vi "Initialize Tasks - NTask.vi"(6 "initialize and close session behavior":T1, 7 "option string":string, 8 "error in":errorcluster, 9 "reset":bool, 11 "session reservation in":refnum<class "Session Reservation.lvclass">) -> (0 "error out":errorcluster, 1 "channel lists":string[](array[string]), 2 "tasks":refnum<class "Session Factory.lvclass">[](array[class]), 3 "session reservation out":refnum<class "Session Reservation.lvclass">)   [LabVIEW 2021, in "Session Management niDAQmx.lvlib"]
uses:
  Session Management niDAQmx.lvlib
  <vilib>/Plug-In SDKs/Clients/Session Management V1/Session Reservation/Initialize and Close Session Behavior.ctl
  <vilib>/Plug-In SDKs/Clients/Session Management V1/Session Reservation/Session Reservation.lvclass
  Session Factory/Session Factory.lvclass
  C:/Program Files/National Instruments/LabVIEW 2021/vi.lib/Plug-In SDKs/Sessions/Instrument/ISession Factory/ISession Factory.lvclass
  22e4e70a-b88f-404f-ac8b-cea03784f9c7.vi
  <vilib>/Plug-In SDKs/Clients/Session Management V1/Session Reservation/Initialize Sessions with Retry.vi
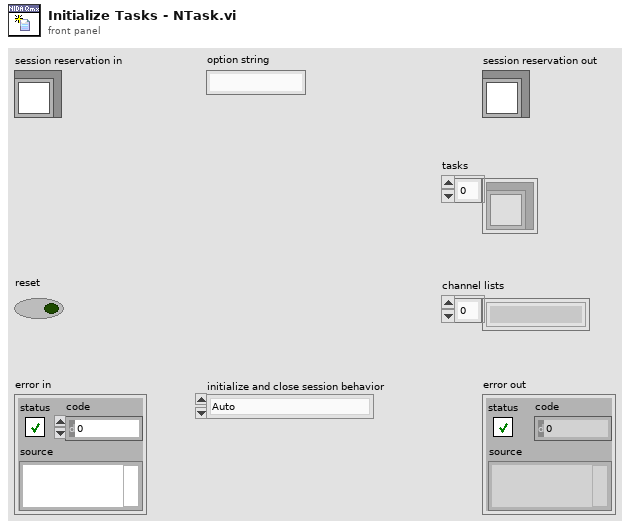
[diagram p1: front panel]
types:
  T1 = typedef "NI Session Management V1 Client.lvlib/Session Reservation.lvclass/Initialize and Close Session Behavior.ctl" = enum16{"Auto", "Initialize and Close", "Attach and Detach", "Initialize and Detach", "Attach and Close"}
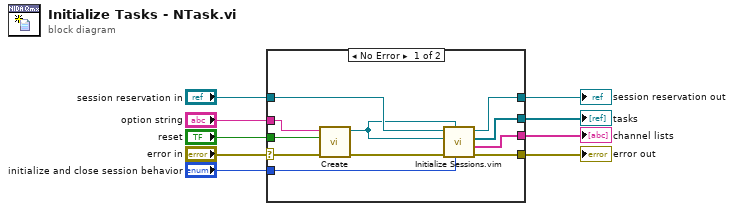
[diagram p0: block diagram]
diagram:
  n1 = case shown="No Error" "error in" {
    selector: "error in" -> [w20 w21]
    tunnel: "session reservation in" -> [w16 w22]
    tunnel: "reset" -> [w18 _]
    tunnel: "option string" -> [w19 _]
    tunnel: "initialize and close session behavior" -> [w15 _]
    tunnel: [w14 w21] -> w3
    tunnel: [w13 w22] -> w4
    tunnel: [w12 _] -> w1
    tunnel: [w11 _] -> w2
    frame No Error {
      n2 = call "Create.vi"("error in"=w20, "reset"=w18, "option string"=w19) -> ("error out"=w17:errorcluster, "session factory out"=w10:refnum<class "Session Factory.lvclass">)  [unwired: 7 in]
      n3 = call "Initialize Sessions.vim"("initialize and close session behavior"=w15, "session type"=w10, "error in"=w17, "session factory"=w10, "session reservation in"=w16) -> ("error out"=w14:errorcluster, "channel lists"=w11:string[], "sessions"=w12:refnum<class "Session Factory.lvclass">[], "session reservation out"=w13:refnum<class "Session Reservation.lvclass">)  [unwired: 3 in]
    }
    frame Error {
    }
  }
  "error out" <- w3
  "session reservation out" <- w4
  "channel lists" <- w2
  "tasks" <- w1
